vi "broadcastTiming.vi"(8 "error in (no error)":errorcluster, 10 "Latency in":u32, 11 "FixedFrameBuilder in":refnum<class "FixedFrameBuilder.lvclass">) -> (0 "error out":errorcluster, 1 "WaitForRxTimeout":u16, 2 "Latency out":u32, 3 "FixedFrameBuilder out":refnum<class "FixedFrameBuilder.lvclass">)   [LabVIEW 2016, in "RTModbus.lvlib" / "FixedFrameBuilder.lvclass"]
uses:
  FixedFrameBuilder.lvclass
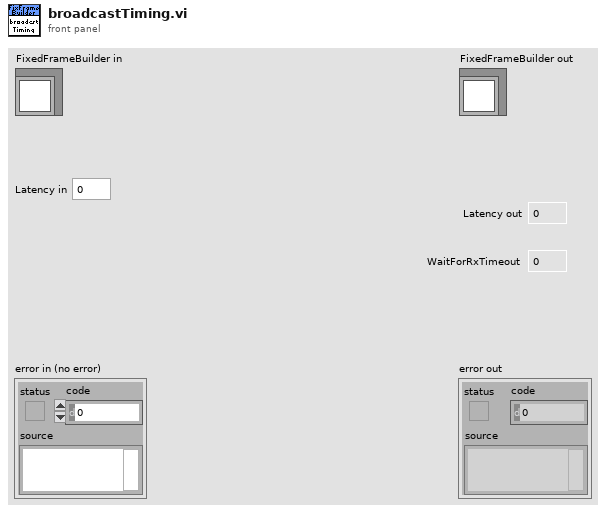
[diagram p1: front panel]
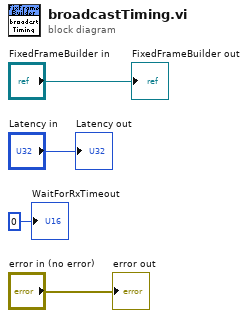
[diagram p0: block diagram]
diagram:
  "error out" <- "error in (no error)"
  "FixedFrameBuilder out" <- "FixedFrameBuilder in"
  "WaitForRxTimeout" <- u16 0 ("WaitForRxTimeout")
  "Latency out" <- "Latency in"
